vi "Init Code String.vi"(0 "Code String in":refnum<class "Code String.lvclass">, 7 "Editable? (T)":bool=TRUE, 11 "error in (no error)":errorcluster) -> (4 "Code String out":refnum<class "Code String.lvclass">, 15 "error out":errorcluster)   [LabVIEW 2016, in "Code String.lvclass"]
doc: "Initializes and displays the Code String panel in the given <b>Subpanel</b>. If <b>Editable?</b> is False, the panel will not be able to be modified through the GUI.\n--------------------\nCopyright (c) 2019 Analog Devices, Inc. All rights reserved.\n\nRedistribution and use in source and binary forms, with or without modification,\nare permitted provided that the following conditions are met:\n - Redistributions of source code must retain the above copyright notice, this\n list of conditions and the following disclaimer.\n - Redistributions in binary form must reproduce the above copyright notice,\n this list of conditions and the following disclaimer in the documentation\n and/or other materials provided with the distribution.\n - Modified versions of the software must be conspicuously marked as such.\n - This software is licensed solely and exclusively for use with\n processors/products manufactured by or for Analog Devices, Inc.\n - This software may not be combined or merged with other code in any manner\n that would cause the software to become subject to terms and conditions\n which differ from those listed here.\n - Neither the name of Analog Devices, Inc. nor the names of its contributors\n may be used to endorse or promote products derived from this software\n without specific prior written permission.\n - The use of this software may or may not infringe the patent rights of one or\n more patent holders. This license does not release you from the requirement\n that you obtain separate licenses from these patent holders to use this\n software.\n\nTHIS SOFTWARE IS PROVIDED BY ANALOG DEVICES, INC. AND CONTRIBUTORS \"AS IS\" AND\nANY EXPRESS OR IMPLIED WARRANTIES, INCLUDING, BUT NOT LIMITED TO,\nNON-INFRINGEMENT, TITLE, MERCHANTABILITY AND FITNESS FOR A PARTICULAR PURPOSE\nARE DISCLAIMED. IN NO EVENT SHALL ANALOG DEVICES, INC. OR CONTRIBUTORS BE LIABLE\nFOR ANY DIRECT, INDIRECT, INCIDENTAL, SPECIAL, EXEMPLARY, PUNITIVE OR\nCONSEQUENTIAL DAMAGES (INCLUDING, BUT NOT LIMITED TO, DAMAGES ARISING OUT OF\nCLAIMS OF INTELLECTUAL PROPERTY RIGHTS INFRINGEMENT; PROCUREMENT OF SUBSTITUTE\nGOODS OR SERVICES; LOSS OF USE, DATA, OR PROFITS; OR BUSINESS INTERRUPTION)\nHOWEVER CAUSED AND ON ANY THEORY OF LIABILITY, WHETHER IN CONTRACT, STRICT\nLIABILITY, OR TORT (INCLUDING NEGLIGENCE OR OTHERWISE) ARISING IN ANY WAY OUT OF\nTHE USE OF THIS SOFTWARE, EVEN IF ADVISED OF THE POSSIBILITY OF SUCH DAMAGE.\n\n2019-01-10-7CBSD SLA"
uses:
  Code String.lvclass
  Code String.lvclass/Code String.ctl
panel:
  # "Copyright (c) 2019 Analog Devices, Inc.  All rights reserved.\n\nRedistribution and use in source and binary forms, with or without modification,\nare permitted provided that the following conditions are met:\n  - Redistributions of source code must retain the above copyright notice, this\n    list of conditions and the following disclaimer.\n  - Redistributions in binary form must reproduce the above copyright notice,\n    this list of conditions and the following disclaimer in the documentation\n    and/or other materials provided with the distribution.\n  - Modified versions of the software must be conspicuously marked as such.\n  - This software is licensed solely and exclusively for use with\n    processors/products manufactured by or for Analog Devices, Inc.\n  - This software may not be combined or merged with other code in any manner\n    that would cause the software to become subject to terms and conditions\n    which differ from those listed here.\n  - Neither the name of Analog Devices, Inc. nor the names of its contributors\n    may be used to endorse or promote products derived from this software\n    without specific prior written permission.\n  - The use of this software may or may not infringe the patent rights of one or\n    more patent holders.  This license does not release you from the requirement\n    that you obtain separate licenses from these patent holders to use this\n    software.\n\nTHIS SOFTWARE IS PROVIDED BY ANALOG DEVICES, INC. AND CONTRIBUTORS \"AS IS\" AND\nANY EXPRESS OR IMPLIED WARRANTIES, INCLUDING, BUT NOT LIMITED TO,\nNON-INFRINGEMENT, TITLE, MERCHANTABILITY AND FITNESS FOR A PARTICULAR PURPOSE\nARE DISCLAIMED. IN NO EVENT SHALL ANALOG DEVICES, INC. OR CONTRIBUTORS BE LIABLE\nFOR ANY DIRECT, INDIRECT, INCIDENTAL, SPECIAL, EXEMPLARY, PUNITIVE OR\nCONSEQUENTIAL DAMAGES (INCLUDING, BUT NOT LIMITED TO, DAMAGES ARISING OUT OF\nCLAIMS OF INTELLECTUAL PROPERTY RIGHTS INFRINGEMENT; PROCUREMENT OF SUBSTITUTE\nGOODS OR SERVICES; LOSS OF USE, DATA, OR PROFITS; OR BUSINESS INTERRUPTION)\nHOWEVER CAUSED AND ON ANY THEORY OF LIABILITY, WHETHER IN CONTRACT, STRICT\nLIABILITY, OR TORT (INCLUDING NEGLIGENCE OR OTHERWISE) ARISING IN ANY WAY OUT OF\nTHE USE OF THIS SOFTWARE, EVEN IF ADVISED OF THE POSSIBILITY OF SUCH DAMAGE.\n\n2019-01-10-7CBSD SLA"
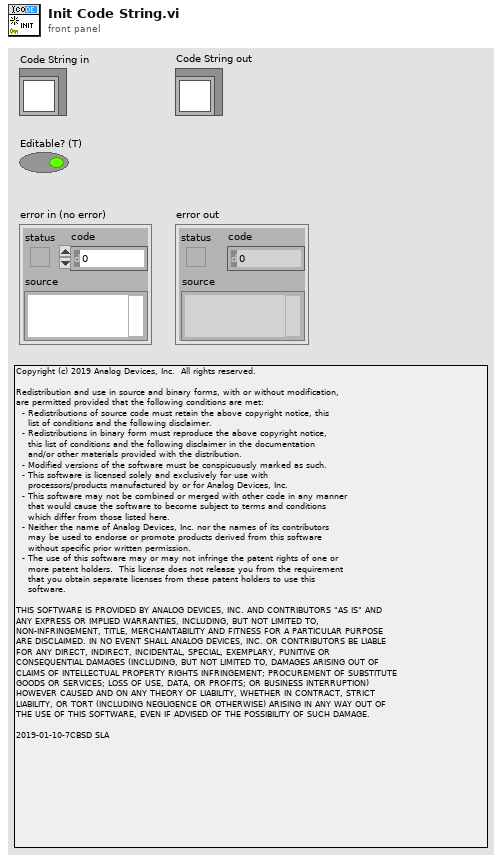
[diagram p1: front panel]
types:
  T1 = typedef "Rendezvous RefNum" = refnum<k1>
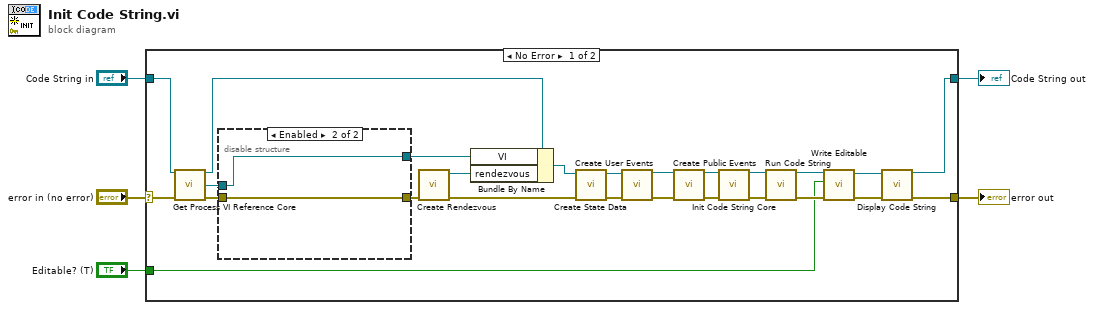
[diagram p0: block diagram]
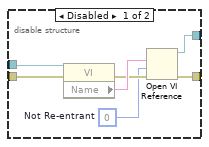
[diagram p2: hidden frame]
diagram:
  n1 = case shown="No Error" "error in (no error)" {
    selector: "error in (no error)" -> [w12 w41]
    tunnel: [w21 w41] -> w4
    tunnel: [w20 w40] -> w2
    tunnel: "Code String in" -> [w9 w40]
    tunnel: "Editable? (T)" -> [w17 _]
    frame No Error {
      n2 = call-dynamic "Get Process VI Reference Core.vi"("Code String in"=w9, "error in (no error)"=w12) -> ("Code String out"=w8:refnum<class "Code String.lvclass">, "Process VI"=w10:refnum<vi>, "error out"=w11:errorcluster)  [unwired: 11 in]
      n3 = disable-structure shown="Enabled" {
        disable-tunnel: [w35 w39] -> w30
        disable-tunnel: [w34 w38] -> w29
        disable-tunnel: w11 -> [w32 w38]
        disable-tunnel: w10 -> [w31 w39]
        frame Disabled {
          w33 = 0  # Not Re-entrant
          n4 = property class="VI"(reference=w31, error in=w32) -> (error out=w36:errorcluster, "Name"=w37:string)  [unwired: 1 out]
          n5 = Open VI Reference(vi path=w37, options=w33, error in (no error)=w36) -> (vi reference=w35:refnum<vi>, error out=w34:errorcluster)  [unwired: 3 in]
        }
        frame Enabled {
        }
      }
      n6 = call <vilib>:"Create Rendezvous.vi"("error in (no error)"=w29) -> ("error out"=w28:errorcluster, "rendezvous"=w27:T1)  [unwired: 4 in, 1 out]
      n7 = Bundle By Name(cluster=w8, "VI"=w30, "rendezvous"=w27) -> (w25:refnum<class "Code String.lvclass">)
      n8 = call "Create State Data.vi"("error in (no error)"=w28, "Code String in"=w25) -> ("error out"=w26:errorcluster, "Code String out"=w23:refnum<class "Code String.lvclass">)  [unwired: 8 in]
      n9 = call "Create User Events.vi"("Code String in"=w23, "error in (no error)"=w26) -> ("Code String out"=w14:refnum<class "Code String.lvclass">, "error out"=w24:errorcluster)  [unwired: 12 in]
      n10 = call "Create Public Events.vi"("Code String in"=w14, "error in (no error)"=w24) -> ("Code String out"=w13:refnum<class "Code String.lvclass">, "error out"=w15:errorcluster)  [unwired: 12 in]
      n11 = call-dynamic "Init Code String Core.vi"("Code String in"=w13, "error in (no error)"=w15) -> ("Code String out"=w6:refnum<class "Code String.lvclass">, "error out"=w7:errorcluster)  [unwired: 12 in]
      n12 = call "Run Code String.vi"("Code String in"=w6, "error in (no error)"=w7) -> ("Code String out"=w18:refnum<class "Code String.lvclass">, "error out"=w22:errorcluster)  [unwired: 12 in]
      n13 = call "Write Editable.vi"("error in (no error)"=w22, "Editable"=w17, "Code String in"=w18) -> ("error out"=w19:errorcluster, "Code String out"=w16:refnum<class "Code String.lvclass">)  [unwired: 7 in]
      n14 = call "Display Code String.vi"("Code String in"=w16, "error in (no error)"=w19) -> ("Code String out"=w20:refnum<class "Code String.lvclass">, "error out"=w21:errorcluster)  [unwired: 12 in]
    }
    frame Error {
    }
  }
  "error out" <- w4
  "Code String out" <- w2
